vi "TestDataFlow.vi"() -> ()   [LabVIEW 2017]
uses:
  <vilib>/addons/Qbus/Qbus.lvclass
  <vilib>/addons/InsightCM/Devices/Shared/Common/ServerComm/ServerComm.lvlib
  <vilib>/NI/Software Watchdog/Pound/Pound.lvclass
  <vilib>/addons/TimerProcess/TimerProcess.lvlib
  <vilib>/addons/Qbus/controls/state.ctl
  <vilib>/addons/InsightCM/Devices/Shared/Common/DataFlow/test/SpeedBenchmark/Loop1/Loop1.lvlib
  <vilib>/addons/InsightCM/Devices/Shared/Common/DataFlow/test/SpeedBenchmark/Loop2/Loop2.lvlib
  <vilib>/addons/InsightCM/Devices/Shared/Common/DataFlow/test/SpeedBenchmark/Loop3/Loop3.lvlib
  <vilib>/addons/InsightCM/Devices/Shared/Common/DataFlow/test/SpeedBenchmark/Loop4/Loop4.lvlib
  <vilib>/addons/InsightCM/Devices/Shared/Common/DataFlow/test/SpeedBenchmark/Loop5/Loop5.lvlib
  <vilib>/addons/InsightCM/Devices/Shared/Common/DataFlow/test/SpeedBenchmark/Loop6/Loop6.lvlib
  <vilib>/addons/InsightCM/Devices/Shared/Common/DataFlow/test/SpeedBenchmark/Loop7/Loop7.lvlib
  <vilib>/addons/InsightCM/Devices/Shared/Common/DataFlow/test/SpeedBenchmark/Loop8/Loop8.lvlib
  <vilib>/addons/InsightCM/Devices/Shared/Common/DataFlow/test/SpeedBenchmark/Loop9/Loop9.lvlib
  <vilib>/addons/InsightCM/Devices/Shared/Common/DataFlow/test/SpeedBenchmark/Loop10/Loop10.lvlib
  <vilib>/addons/InsightCM/MessageBus/Base/controls/ConnectionInfo.ctl
panel:
  out "per message":dbl format="%#_6e"
  out "execution time":dbl
  out "error out":errorcluster
  out "Listbox":i32(listbox)
  in  "ConnInfo":T1={"ClientName"="Bop9068", "TransceiverHost"="10.2.64.56", "TransceiverPort"=6342, "Password"="password"}
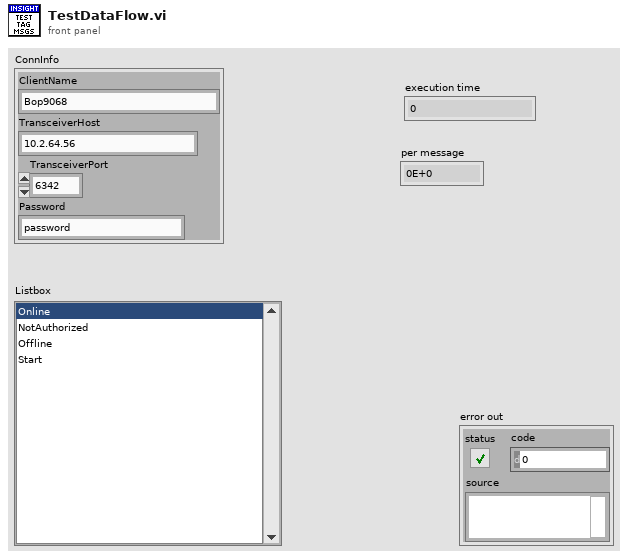
[diagram p1: front panel]
types:
  T1 = typedef "ConnectionInfo.ctl" = cluster{"ClientName":string, "TransceiverHost":string, "TransceiverPort":u16, "Password":string}
  T2 = typedef "Qbus.lvclass/state.ctl" = enum16{"unconfigured", "configured"}
  T3 = typedef "ServerComm.lvlib/ConnectionStatus.ctl" = enum16{"Offline", "NotAuthorized", "Online"}
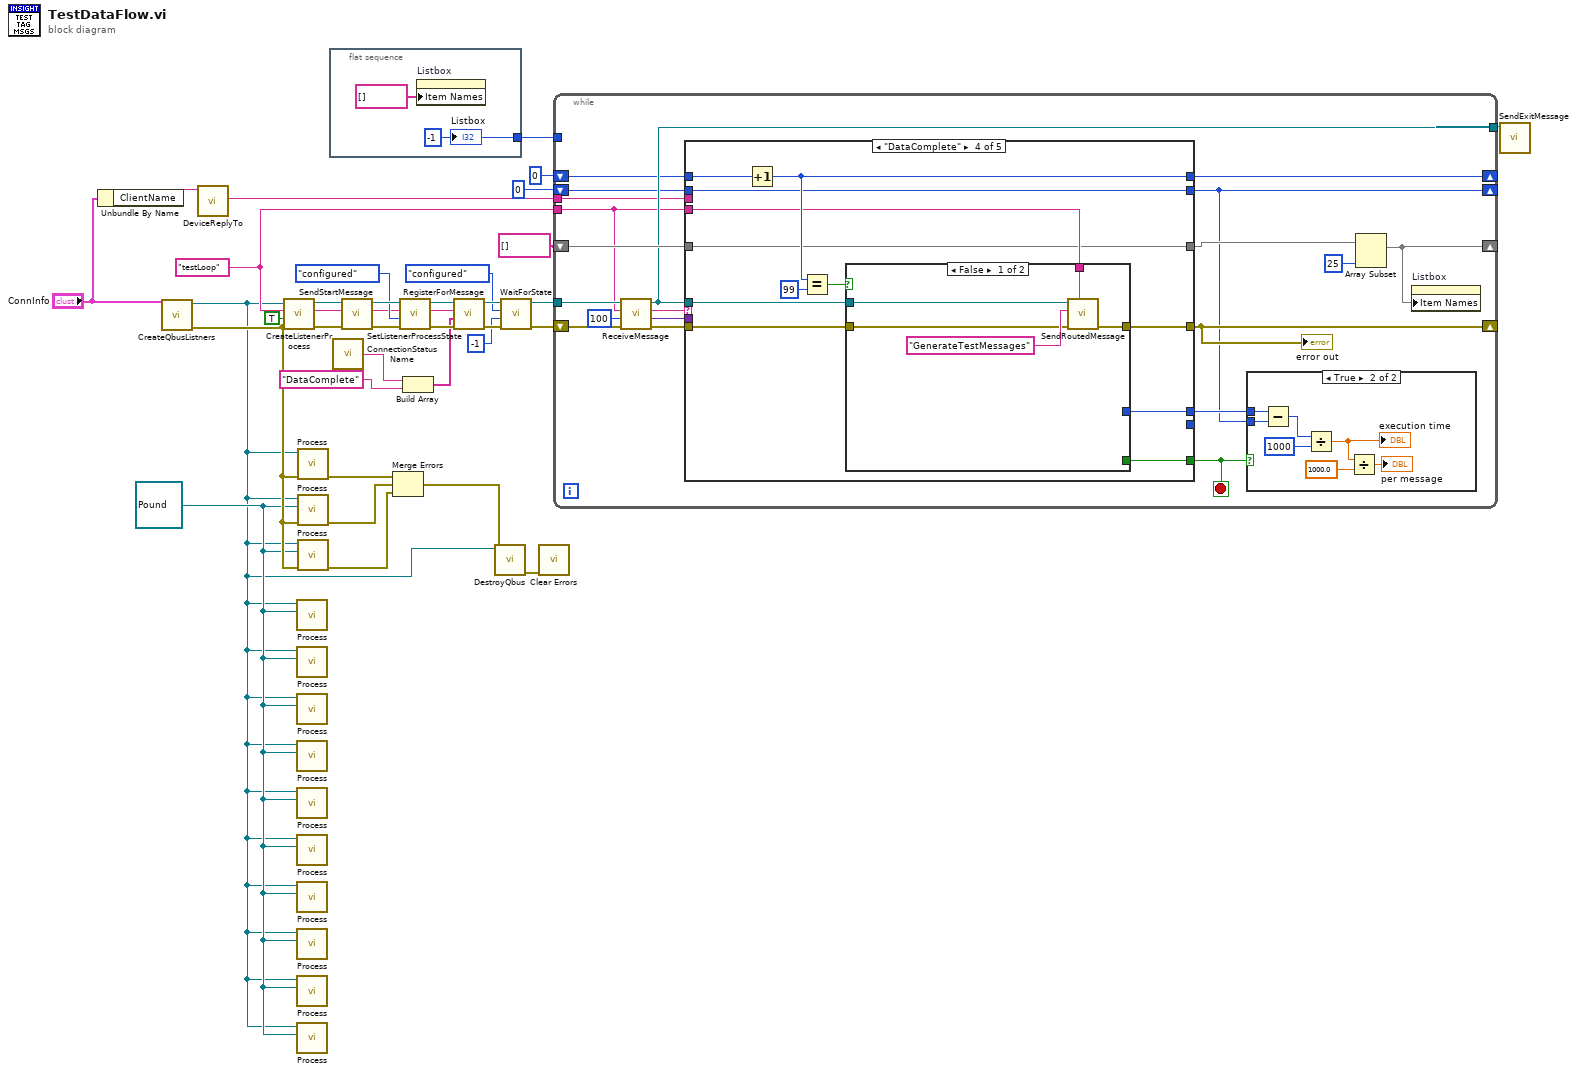
[diagram p0: block diagram]
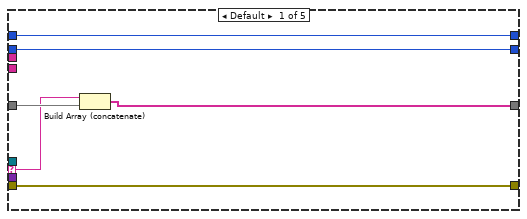
[diagram p3: hidden frame]
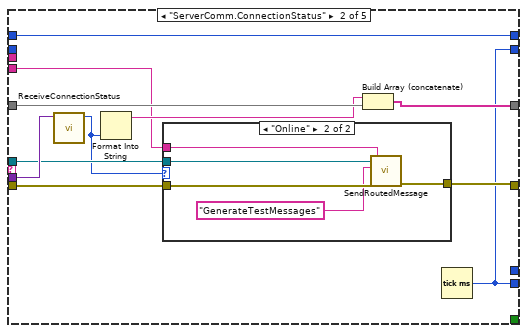
[diagram p4: hidden frame]
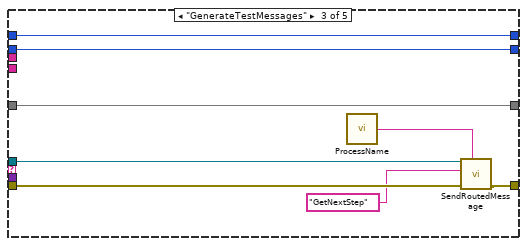
[diagram p6: hidden frame]
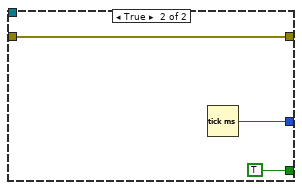
[diagram p7: hidden frame]
diagram:
  w4 = refnum<class "Pound.lvclass"> refnum ("Pound in")
  w8 = "testLoop" ("ProcessName")
  n1 = Unbundle By Name("ConnInfo") -> ("ClientName"=w7:string)
  n2 = call <vilib>:"CreateQbusListners.vi"("ConnInfo"="ConnInfo") -> ("error out"=w5:errorcluster, "Qbus out"=w3:refnum<class "Qbus.lvclass">)  [unwired: 9 in]
  n3 = call <vilib>:"DeviceReplyTo.vi"("Device"=w7) -> ("ReplyTo"=w6:string)  [unwired: 10 in]
  n4 = call <vilib>:"CreateListenerProcess.vi"("error in (no error)"=w5, "master"=TRUE ("Master"), "process name"=w8, "Qbus in"=w3) -> ("error in (no error)"=w31:errorcluster, "Qbus out"=w34:refnum<class "Qbus.lvclass">)  [unwired: 6 in]
  n5 = call <vilib>:"Process.vi"("Pound in"=w4, "Qbus in"=w3) -> ()  [unwired: 9 in, 1 out]
  n6 = call <vilib>:"Process.vi"("Pound in"=w4, "Qbus in"=w3) -> ()  [unwired: 9 in, 1 out]
  n7 = call <vilib>:"Process.vi"("Pound in"=w4, "Qbus in"=w3) -> ()  [unwired: 9 in, 1 out]
  n8 = call <vilib>:"Process.vi"("Pound in"=w4, "Qbus in"=w3) -> ()  [unwired: 9 in, 1 out]
  n9 = call <vilib>:"Process.vi"("Pound in"=w4, "Qbus in"=w3) -> ()  [unwired: 9 in, 1 out]
  n10 = call <vilib>:"Process.vi"("Pound in"=w4, "Qbus in"=w3) -> ()  [unwired: 9 in, 1 out]
  n11 = call <vilib>:"Process.vi"("Pound in"=w4, "Qbus in"=w3) -> ()  [unwired: 9 in, 1 out]
  n12 = call <vilib>:"Process.vi"("Pound in"=w4, "Qbus in"=w3) -> ()  [unwired: 9 in, 1 out]
  n13 = call <vilib>:"Process.vi"("Pound in"=w4, "Qbus in"=w3) -> ()  [unwired: 9 in, 1 out]
  n14 = call <vilib>:"Process.vi"("Pound in"=w4, "Qbus in"=w3) -> ()  [unwired: 9 in, 1 out]
  n15 = call <vilib>:"Process.vi"("error in (no error)"=w5, "Qbus in"=w3) -> ("error out"=w29:errorcluster)  [unwired: 9 in]
  n16 = call <vilib>:"Process.vi"("error in (no error)"=w5, "Pound in"=w4, "Qbus in"=w3) -> ("error out"=w27:errorcluster)  [unwired: 8 in]
  n17 = call <vilib>:"Process.vi"("error in (no error)"=w5, "pound in"=w4, "qbus in"=w3) -> ("error out"=w19:errorcluster)  [unwired: 8 in]
  n18 = flat-sequence {
    tunnel: [w36] -> w10
    frame #0 {
      w36 = -1 ("Listbox")
      n19 = property on="Listbox" class="LstBox (strict)"("Item Names"=string[] []) -> ()  [unwired: 2 in, 2 out]
      "Listbox" <- w36
    }
  }
  n20 = call <vilib>:"ConnectionStatusName.vi"() -> ("message name"=w20:string)  [unwired: 5 in]
  n21 = call <vilib>:"SendStartMessage.vi"("error in (no error)"=w31, "Qbus in"=w34) -> ("error out"=w32:errorcluster, "Qbus out"=w33:refnum<class "Qbus.lvclass">)  [unwired: 8 in]
  n22 = Merge Errors(w29, w27, w19) -> (w28:errorcluster)
  n23 = call <vilib>:"SetListenerProcessState.vi"("error in (no error)"=w32, "state"=state."configured", "ProcessName"=w8, "Qbus in"=w33) -> ("error out"=w22:errorcluster, "Qbus out"=w23:refnum<class "Qbus.lvclass">)  [unwired: 6 in]
  n24 = Build Array(w20, "DataComplete" ("MsgName")) -> (w21:string[])
  n25 = call <vilib>:"RegisterForMessage.vi"("error in (no error)"=w22, "message names"=w21, "process name"=w8, "Qbus in"=w23) -> ("error in (no error)"=w16:errorcluster, "Qbus out"=w17:refnum<class "Qbus.lvclass">)  [unwired: 6 in]
  n26 = call <vilib>:"DestroyQbus.vi"("error in (no error)"=w28, "Qbus"=w3) -> ("error in (no error)"=w24:errorcluster)  [unwired: 9 in]
  n27 = call <vilib>:"WaitForState.vi"("error in (no error)"=w16, "timeout (-1)"=-1, "state"=state."configured", "Qbus in"=w17) -> ("error out"=w15:errorcluster, "Qbus out"=w14:refnum<class "Qbus.lvclass">)  [unwired: 4 in, 2 out]
  n28 = call <vilib>:"Clear Errors.vi"("error in (no error)"=w24) -> ()  [unwired: 5 in, 2 out]
  n29 = while {
    tunnel: w14 -> [w56]
    tunnel: w6 -> [w44]
    tunnel: [w47] -> w26
    shift-right: [w49] -> _
    shift-left: string[] [] -> [w52]
    shift-right: [w45] -> _
    shift-left: w15 -> [w55]
    tunnel: w10 -> [_]
    tunnel: w8 -> [w43]
    shift-right: [w40] -> _
    shift-left: 0 -> [w42]
    shift-right: [w38] -> _
    shift-left: u32 0 ("millisecond timer value") -> [w39]
    stop <- w37 stop-if-true
    n30 = call <vilib>:"ReceiveMessage.vi"("error in (no error)"=w55, "timeout (0)"=100, "process name"=w43, "Qbus in"=w56) -> ("error in (no error)"=w46:errorcluster, "message value"=w48:variant, "message name"=w53:string, "Qbus out"=w47:refnum<class "Qbus.lvclass">)  [unwired: 2 in, 2 out]
    n31 = case shown="\"DataComplete\"" w53 {
      selector: w53 -> [w68 _ _ _ _]
      tunnel: [w67 w79 w88 w96 w118] -> w50
      tunnel: w52 -> [w69 w80 w88 w96 w118]
      tunnel: w48 -> [_ w77 _ _ _]
      tunnel: w47 -> [_ w76 w92 w99 _]
      tunnel: w46 -> [w66 w75 w93 w102 w117]
      tunnel: [w66 w74 w94 w101 w117] -> w45
      tunnel: w44 -> [_ _ _ _ _]
      tunnel: w43 -> [_ w72 _ w98 _]
      tunnel: [w65 w71 w89 w105 w116] -> w40
      tunnel: w42 -> [w65 w71 w89 w106 w116]
      tunnel: [_ _ _ w100 _] -> w41
      tunnel: [_ w70 _ _ _] -> _
      tunnel: [_ _ _ w97 _] -> w37
      tunnel: [w64 w70 w87 w95 w115] -> w38
      tunnel: w39 -> [w64 _ w87 w95 w115]
      frame Default {
        n32 = Build Array (concatenate)(w68, w69) -> (w67:string[])
      }
      frame "ServerComm.ConnectionStatus" {
        n33 = call <vilib>:"ReceiveConnectionStatus.vi"("body"=w77) -> ("status"=w73:T3)  [unwired: 7 in, 3 out]
        n34 = Format Into String(w73) -> (resulting string=w78:string)  [unwired: 3 in, 1 out]
        n35 = case shown="\"Online\"" w73 {
          tunnel: w76 -> [_ w86]
          tunnel: w75 -> [w81 w85]
          tunnel: [w81 w84] -> w74
          tunnel: w72 -> [_ w82]
          frame "Offline", Default {
          }
          frame "Online" {
            n36 = call <vilib>:"SendRoutedMessage.vi"("listener process"=w82, "error in (no error)"=w85, "message name"="GenerateTestMessages" ("MsgName"), "Qbus in"=w86) -> ("error in (no error)"=w84:errorcluster)  [unwired: 6 in, 1 out]
          }
        }
        n37 = Build Array (concatenate)(w78, w80) -> (w79:string[])
        n38 = Tick Count (ms)() -> (millisecond timer value=w70:u32)
      }
      frame "GenerateTestMessages" {
        n39 = call <vilib>:"ProcessName.vi"() -> ("ProcessName"=w90:string)  [unwired: 5 in]
        n40 = call <vilib>:"SendRoutedMessage.vi"("listener process"=w90, "error in (no error)"=w93, "message name"="GetNextStep", "Qbus in"=w92) -> ("error in (no error)"=w94:errorcluster)  [unwired: 6 in, 1 out]
      }
      frame "DataComplete" {
        n41 = Increment(x=w106) -> (x+1=w105:i32)
        n42 = Equal?(x=w105, y=99) -> (x = y?=w103:bool)
        n43 = case shown="False" w103 {
          tunnel: w102 -> [w110 w114]
          tunnel: [w109 w114] -> w101
          tunnel: [_ w113] -> w100
          tunnel: w99 -> [w108 _]
          tunnel: w98 -> [w107 _]
          tunnel: [_ TRUE] -> w97
          frame False {
            n44 = call <vilib>:"SendRoutedMessage.vi"("listener process"=w107, "error in (no error)"=w110, "message name"="GenerateTestMessages" ("MsgName"), "Qbus in"=w108) -> ("error in (no error)"=w109:errorcluster)  [unwired: 6 in, 1 out]
          }
          frame True {
            n45 = Tick Count (ms)() -> (millisecond timer value=w113:u32)
          }
        }
      }
      frame "" {
      }
    }
    "error out" <- w45
    n46 = case shown="True" w37 {
      tunnel: w41 -> [_ w63]
      tunnel: w38 -> [_ w60]
      frame False {
      }
      frame True {
        n47 = Subtract(x=w63, y=w60) -> (x-y=w62:u32)
        n48 = Divide(x=w62, y=u32 1000) -> (x/y=w59:dbl)
        "execution time" <- w59
        n49 = Divide(x=w59, y=1000.0) -> (x/y=→"per message":dbl)
      }
    }
    n50 = Array Subset(array=w50, length=25) -> (w49:string[])  [unwired: 1 in]
    n51 = property on="Listbox" class="LstBox (strict)"("Item Names"=w49) -> ()  [unwired: 2 in, 2 out]
  }
  n52 = call <vilib>:"SendExitMessage.vi"("Qbus in"=w26) -> ()  [unwired: 9 in, 2 out]
